vi "InitTempTableTlog.vi"(6 "AllYData In":dbl[][](array[numeric]), 7 "TousTemps In":dbl[](array[numeric]), 8 "error in (no error)":errorcluster, 9 "nb de courbe":i32=9, 10 "Max de Points":i32=84600, 11 "Clear Ref":refnum<vi>) -> (0 "error out":errorcluster, 4 "AllYData":dbl[][](array[numeric]), 5 "TousTemps":dbl[](array[numeric]))   [LabVIEW 2010]
doc: "Ce Vi initialise les tableaux de temps et de données d'acquisitions à la dimensions voulu."
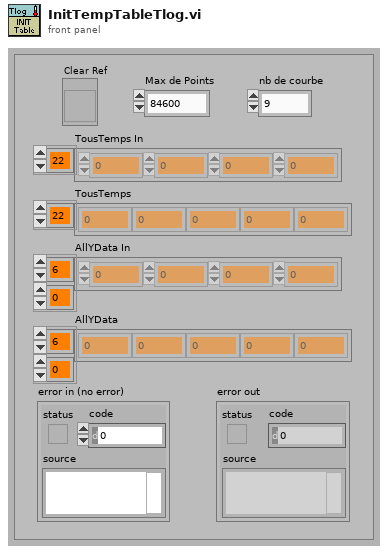
[diagram p1: front panel]
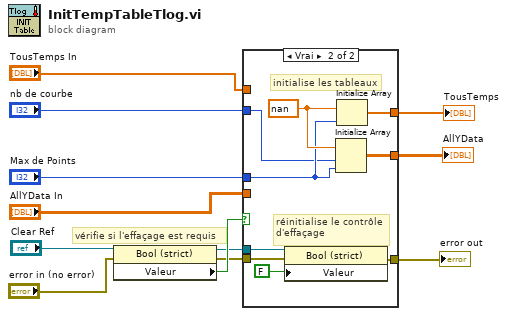
[diagram p0: block diagram]
diagram:
  # "vérifie si l'effaçage est requis"
  n1 = property class="Bool (strict)"(reference="Clear Ref", error in="error in (no error)") -> (reference out=w3:refnum<vi>, error out=w2:errorcluster, "Valeur"=w5:bool)
  n2 = case shown="Vrai" w5 {
    tunnel: "Max de Points" -> [_ w23]
    tunnel: "nb de courbe" -> [_ w22]
    tunnel: [w14 w21] -> w10
    tunnel: [w15 w20] -> w9
    tunnel: "AllYData In" -> [w14 _]
    tunnel: "TousTemps In" -> [w15 _]
    tunnel: w3 -> [_ w19]
    tunnel: w2 -> [w13 w18]
    tunnel: [w13 w16] -> w1
    frame False {
    }
    frame True {
      w24 = nan ("element")
      # "initialise les tableaux"
      # "réinitialise le contrôle\nd'effaçage"
      n3 = property class="Bool (strict)"(reference=w19, error in=w18, "Valeur"=FALSE) -> (error out=w16:errorcluster)  [unwired: 1 out]
      n4 = Initialize Array(w24, w22, w23) -> (w21:dbl[][])
      n5 = Initialize Array(w24, w23) -> (w20:dbl[])
    }
  }
  "TousTemps" <- w9
  "AllYData" <- w10
  "error out" <- w1
